vi "emi_Tabs Set Active.vi"(0 "Tab Control":refnum<vi>, 7 "Tab index":u16, 11 "error In":errorcluster) -> (4 "Tab Control Out":refnum<vi>, 15 "error out":errorcluster)   [LabVIEW 2010]
doc: "Set the actrive tab on a tab control, by index number(0..)\n\nOn error, do nothing"
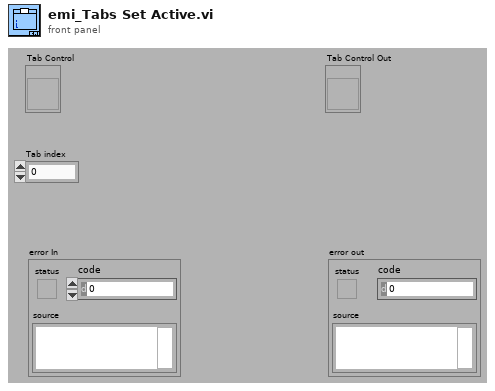
[diagram p1: front panel]
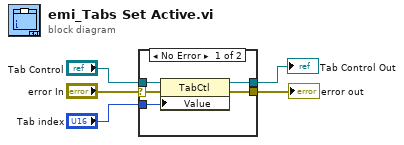
[diagram p0: block diagram]
diagram:
  n1 = case shown="No Error" "error In" {
    selector: "error In" -> [w6 w11]
    tunnel: [w10 w11] -> w5
    tunnel: "Tab Control" -> [w9 w12]
    tunnel: [w8 w12] -> w3
    tunnel: "Tab index" -> [w7 _]
    frame No Error {
      n2 = property class="TabCtl"(reference=w9, error in=w6, "Value"=w7) -> (reference out=w8:refnum<vi>, error out=w10:errorcluster)
    }
    frame Error {
    }
  }
  "error out" <- w5
  "Tab Control Out" <- w3
